vi "SeqMgr.For Loop Compare Values.vi"(8 "error in":errorcluster, 11 "Var,Start,End,Inc":string[](array[string])) -> (0 "error out":errorcluster, 2 "Counter New Val":string, 3 "Continue":bool)   [LabVIEW 2024, in "EQMF.lvlib" / "SeqMgr.lvlib"]
uses:
  SeqMgr.lvlib
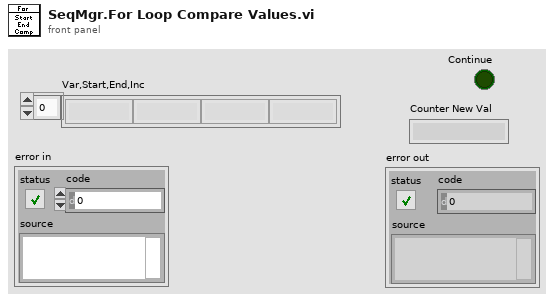
[diagram p1: front panel]
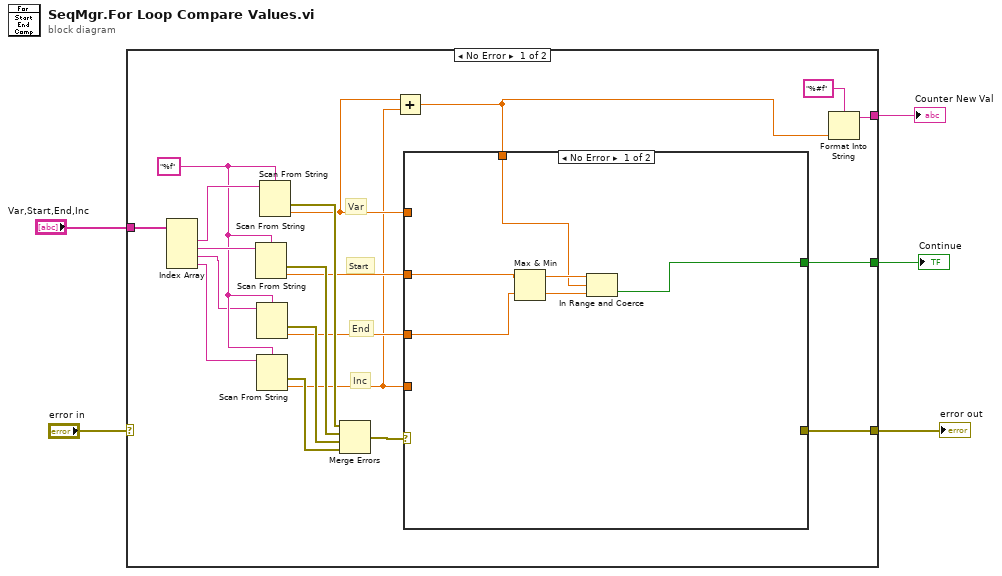
[diagram p0: block diagram]
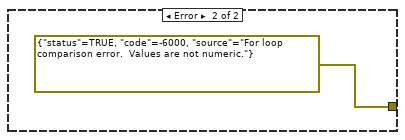
[diagram p2: hidden frame]
diagram:
  n1 = case shown="No Error" "error in" {
    selector: "error in" -> [_ w33]
    tunnel: "Var,Start,End,Inc" -> [w25 _]
    tunnel: [w17 w33] -> w3
    tunnel: [w18 _] -> w2
    tunnel: [w8 _] -> w1
    frame No Error {
      w14 = "%f"
      # "Inc"
      # "End"
      # "Start"
      # "Var"
      n2 = Index Array(array=w25) -> (element #1=w24:string, element #2=w23:string, element #3=w13:string, element #4=w12:string)  [unwired: 4 in]
      n3 = Scan From String(format string=w14, input string=w23) -> (error out=w21:errorcluster, output 1=w19:dbl)  [unwired: 3 in, 2 out]
      n4 = Scan From String(format string=w14, input string=w13) -> (error out=w16:errorcluster, output 1=w11:dbl)  [unwired: 3 in, 2 out]
      n5 = Scan From String(format string=w14, input string=w12) -> (error out=w15:errorcluster, output 1=w9:dbl)  [unwired: 3 in, 2 out]
      n6 = Scan From String(format string=w14, input string=w24) -> (error out=w22:errorcluster, output 1=w10:dbl)  [unwired: 3 in, 2 out]
      n7 = Merge Errors(w22, w21, w16, w15) -> (w20:errorcluster)
      n8 = Add(x=w10, y=w9) -> (x+y=w7:dbl)
      n9 = case shown="No Error" w20 {
        tunnel: w19 -> [w31 _]
        tunnel: w10 -> [_ _]
        tunnel: [w27 _] -> w18
        tunnel: [_ errorcluster {"status"=TRUE, "code"=-6000, "source"="For loop comparison error.  Values are not numeric."} ("error constant")] -> w17
        tunnel: w11 -> [w30 _]
        tunnel: w9 -> [_ _]
        tunnel: w7 -> [w26 _]
        frame No Error {
          n10 = Max & Min(x=w31, y=w30) -> (max(x,y)=w29:dbl, min(x,y)=w28:dbl)
          n11 = In Range and Coerce(upper limit=w29, x=w26, lower limit=w28) -> (In Range?=w27:bool)  [unwired: 1 out]
        }
        frame Error {
        }
      }
      n12 = Format Into String(format string="%#f", w7) -> (resulting string=w8:string)  [unwired: 2 in, 1 out]
    }
    frame Error {
    }
  }
  "Continue" <- w2
  "error out" <- w3
  "Counter New Val" <- w1
